vi "User Interface.vi"(10 "Test File Path":path=path "") -> ()   [LabVIEW 2020, in "Execution UI.lvclass"]
uses:
  Execution UI.lvclass
  Execution UI.lvclass/Execution UI.ctl
  Application Framework/Process Classes/Process/Process.lvclass
  <vilib>/Utility/miscctls.llb/LVNodeAndColumnTypeDef.ctl
  Private/TypeDefs/Execution State.ctl
  Framework/Result View/Result View.vi
  Framework/Test Result View/Test Result View.lvclass
  <vilib>/Platform/browser.llb/Open URL in Default Browser (string).vi
  Core/Result/Status.ctl
  Core/Result/Result.lvlib
  Framework/Result Model/Result Model.lvclass
  Core/Result/Type.ctl
  Core/Result/Result.ctl
  109dbbcd-ccfb-4061-a2e5-43f6d68915f9.vi
  C:/Git/astemes-lunit/source/Application Framework/Process Classes/Process/Process.lvclass
  C:/Git/astemes-lunit/source/Execution UI/Execution UI.lvclass
  C:/Git/astemes-lunit/source/Core/Result Observer/Result Observer.lvclass
panel:
  in  "Refresh":bool
  in  "Run Selected Tests":bool
  in  "Stop":bool
  in  "Run All Tests":bool
  in  "Eject":bool
  in  "Save":bool
  in  "Collapse":bool
  in  "Expand":bool
  out "Progress bar":dbl(slide) scale=0.0..100.0
  out "Results":i32(listbox)=-1
  in  "Test Results":string[](tree)
  in  "Filter fails":bool
  out "Description":string
  out "Status":string
  # "1"
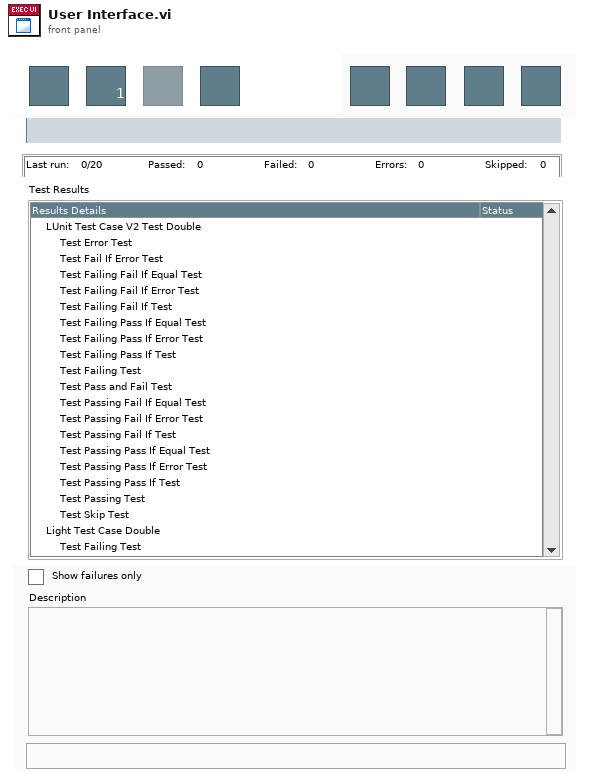
[diagram p1: front panel]
types:
  T1 = typedef "Result Model.lvclass/Statistics.ctl" = cluster{"Method Count":u32, "Executed Methods":u32, "Passed Methods":u32, "Failed Methods":u32, "Method Errors":u32, "Skipped Method":u32, "Progress [%]":dbl}
  T2 = typedef "Execution UI.lvclass/Execution State.ctl" = enum16{"Idle", "Running"}
  T3 = typedef "Result.lvlib/Result.ctl" = cluster{"Name":string, "Message":string, "Description":string, "Status":T4, "Result Type":T5, "Execution Time":dbl}
  T4 = typedef "Result.lvlib/Status.ctl" = enum16{"", "Passed", "Failed", "Error", "Skipped", "Setup Error", "Broken", "Teardown Error"}
  T5 = typedef "Result.lvlib/Type.ctl" = enum16{"Method", "Case", "Suite", "Pass", "Fail", "Skip", "Pass if", "Fail if", "Pass if Error", "Fail if Error", "Pass if Equal", "Fail if Equal"}
  T6 = typedef "LVNodeAndColumnTypeDef.ctl" = cluster{"Node":string, "Column":i32}
  T7 = enum8{"Enabled", "Disabled", "Disabled and Grayed Out"}
  T8 = enum32{"Invalid", "Standard", "Closed", "Hidden", "Minimized", "Maximized"}
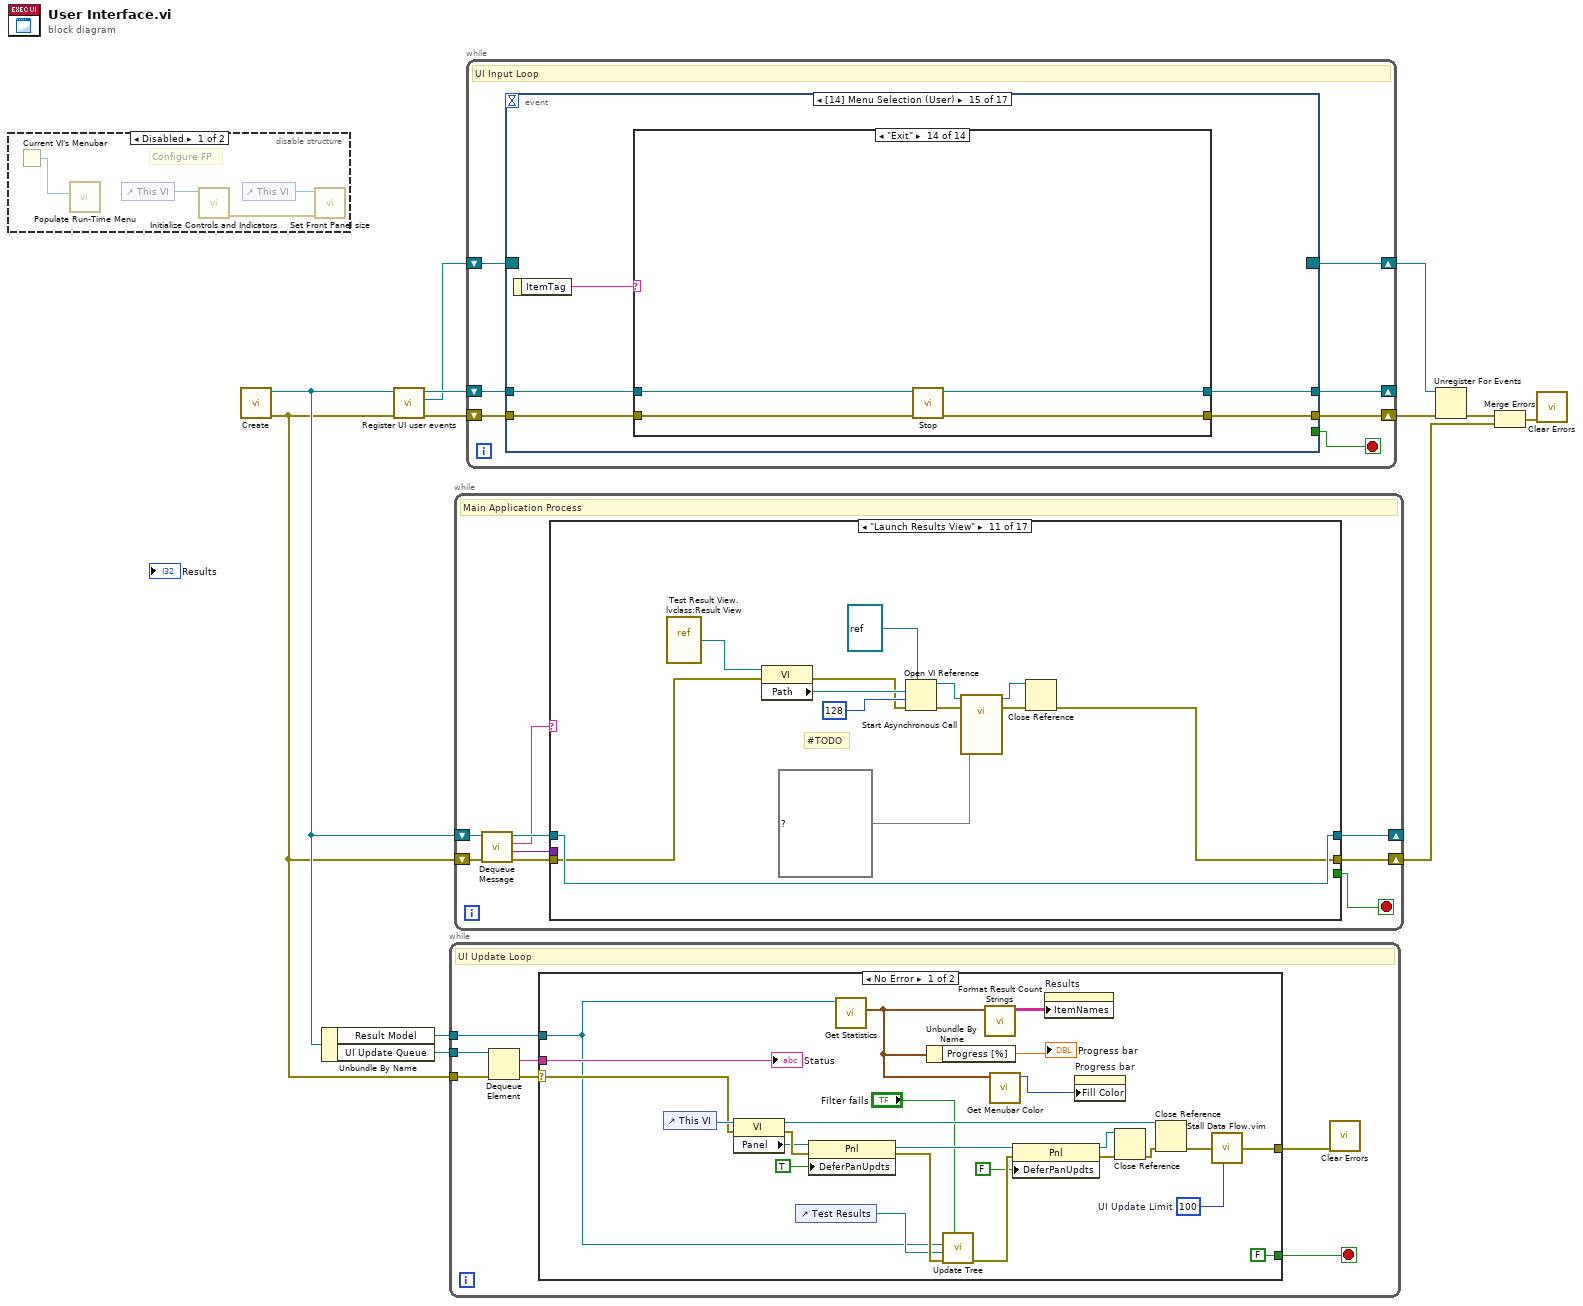
[diagram p0: block diagram]
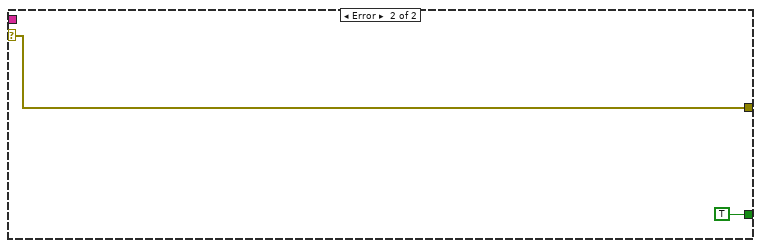
[diagram p2: hidden frame]
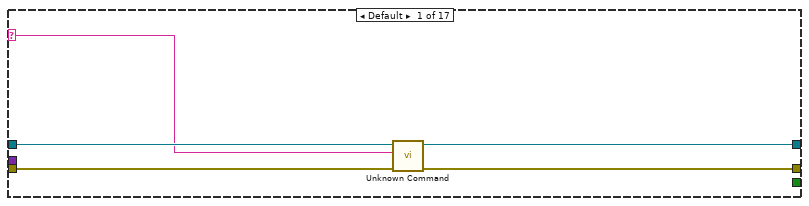
[diagram p3: hidden frame]
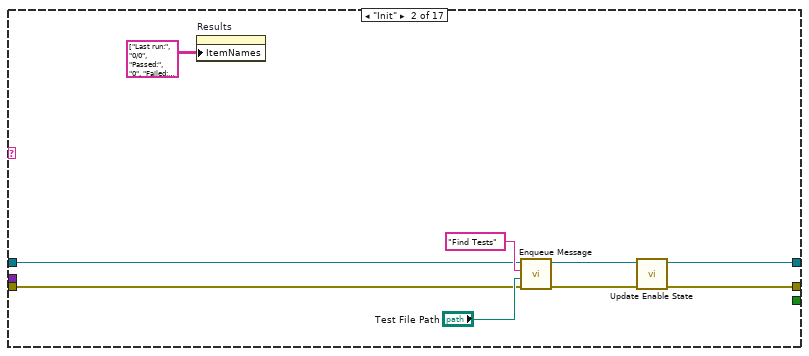
[diagram p4: hidden frame]
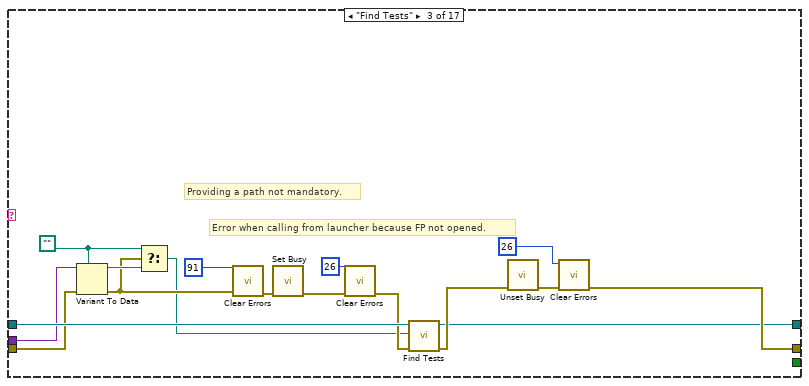
[diagram p5: hidden frame]
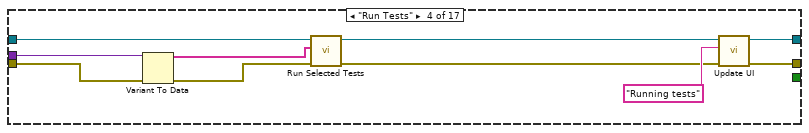
[diagram p6: hidden frame]
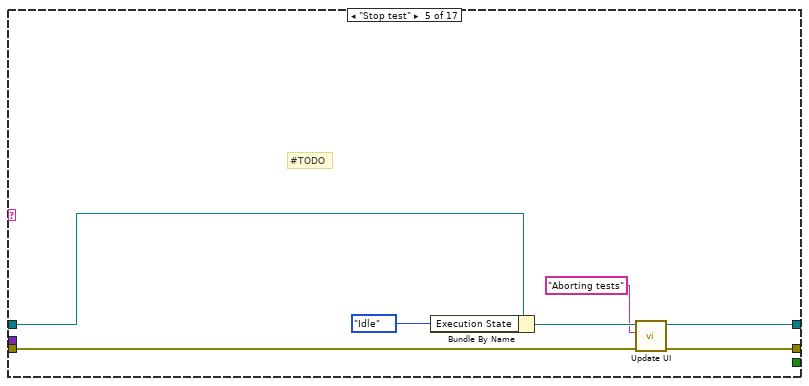
[diagram p7: hidden frame]
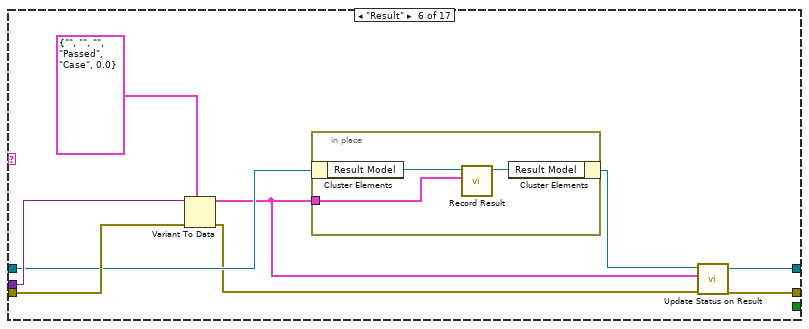
[diagram p8: hidden frame]
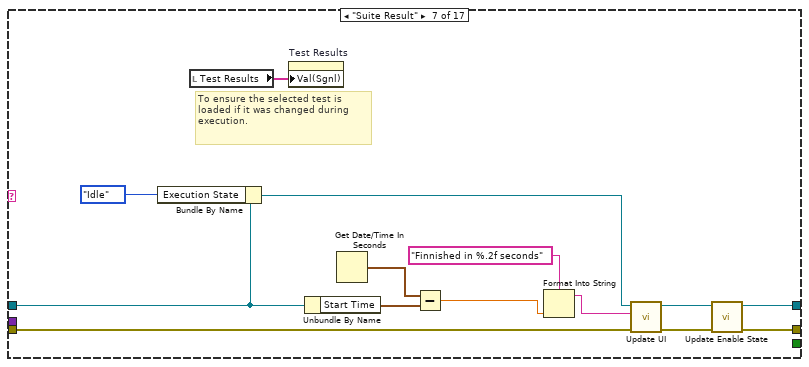
[diagram p9: hidden frame]
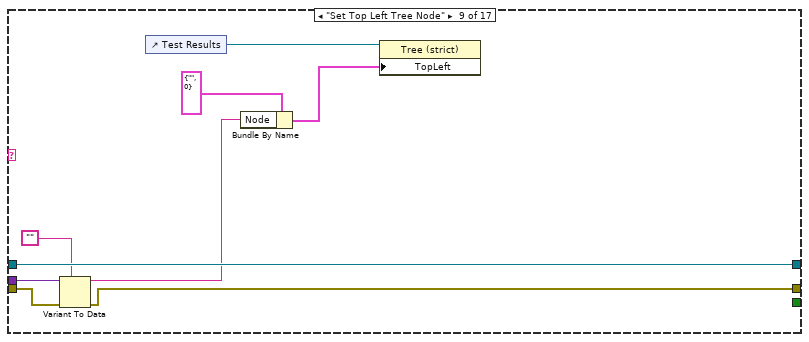
[diagram p11: hidden frame]
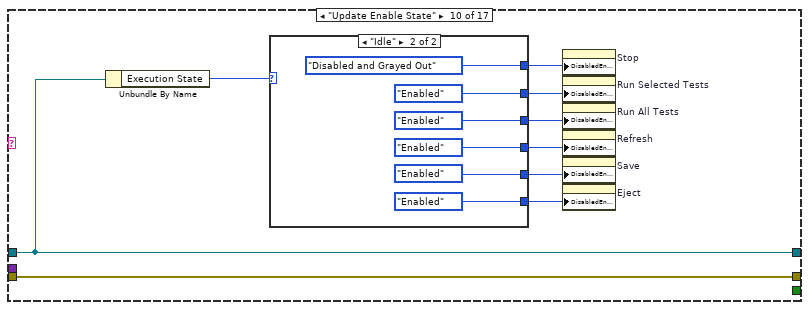
[diagram p12: hidden frame]
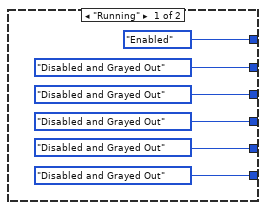
[diagram p13: hidden frame]
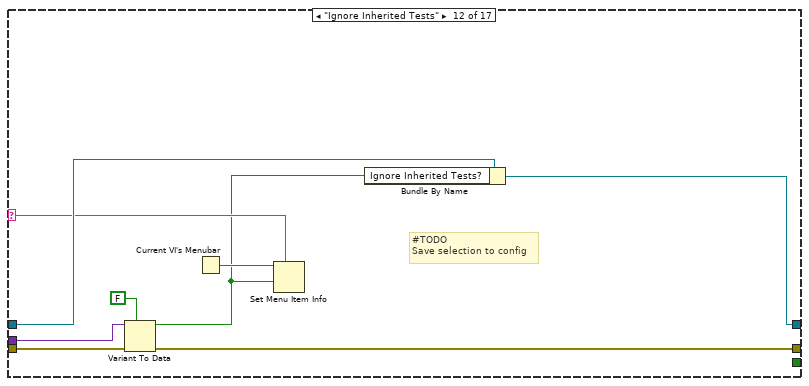
[diagram p14: hidden frame]
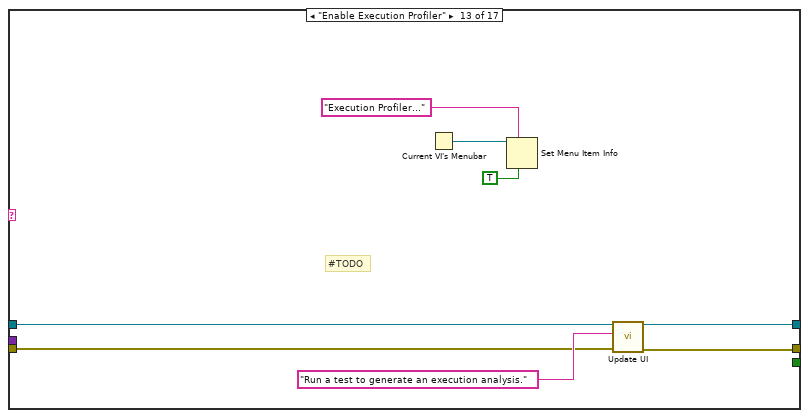
[diagram p15: hidden frame]
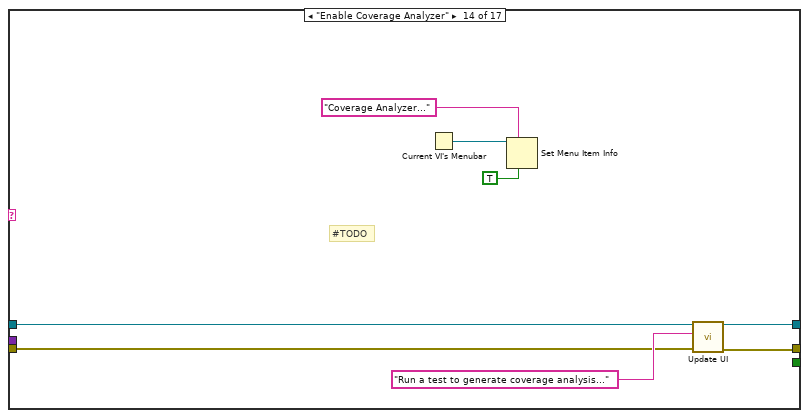
[diagram p16: hidden frame]
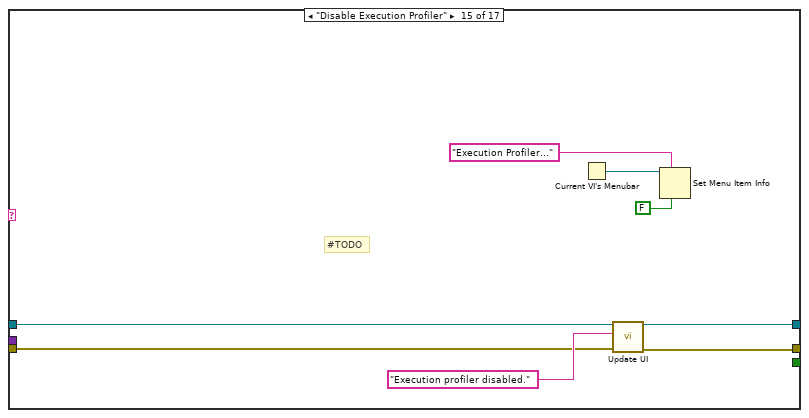
[diagram p17: hidden frame]
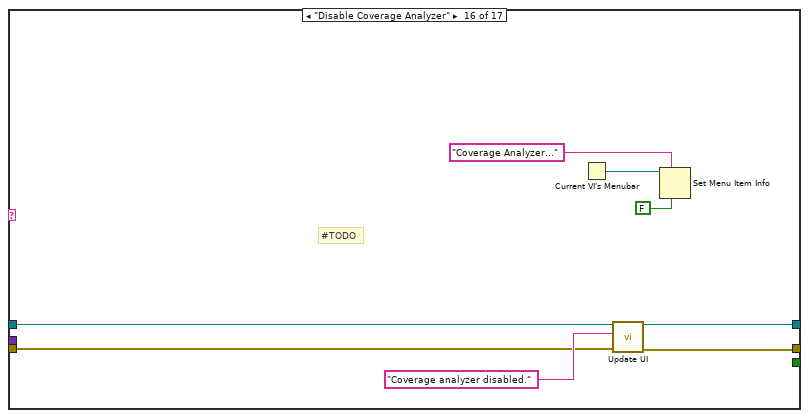
[diagram p18: hidden frame]
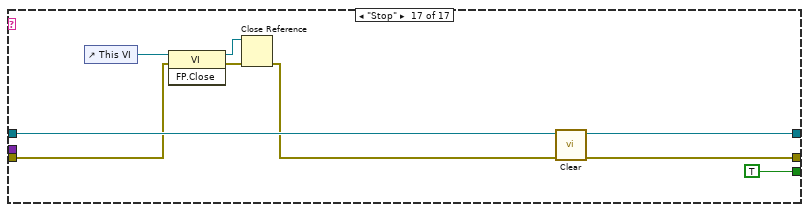
[diagram p19: hidden frame]
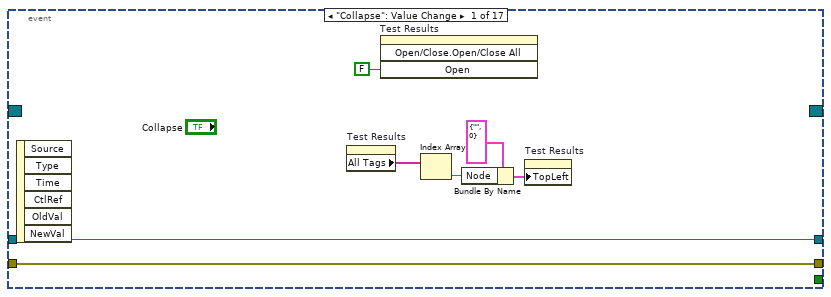
[diagram p20: hidden frame]
diagram:
  n1 = disable-structure shown="Disabled" {
    frame Disabled {
      # "Configure FP"
      n2 = Current VI's Menubar() -> (w13:refnum<k9>)
      n3 = call "Populate Run-Time Menu.vi"("Menu in"=w13) -> ()  [unwired: 9 in, 2 out]
      n4 = control-ref of="This VI"() -> (w15:refnum<vi>)
      n5 = call "Initialize Controls and Indicators.vi"("VI in"=w15) -> ("error out"=w14:errorcluster)  [unwired: 10 in]
      n6 = control-ref of="This VI"() -> (w16:refnum<vi>)
      n7 = call "Set Front Panel size.vi"("error in (no error)"=w14, "VI in"=w16) -> ()  [unwired: 9 in, 1 out]
    }
    frame Enabled {
    }
  }
  n8 = call "Create.vi"() -> ("error out"=w3:errorcluster, "Execution UI Out"=w4:refnum<class "Execution UI.lvclass">)  [unwired: 10 in]
  n9 = Unbundle By Name(w4) -> ("Result Model"=w2:refnum<class "Result Model.lvclass">, "UI Update Queue"=w1:refnum<queue>)
  n10 = call "Register UI user events.vi"("error in (no error)"=w3, "Execution UI In"=w4) -> ("error out"=w11:errorcluster, "Event Registration Refnum"=w9:refnum<event-registration>, "Execution UI Out"=w12:refnum<class "Execution UI.lvclass">)  [unwired: 7 in]
  n11 = while {
    tunnel: w3 -> [w21]
    tunnel: w2 -> [w19]
    tunnel: w1 -> [w18]
    stop <- w17 stop-if-true
    # "UI Update Loop"
    n12 = Dequeue Element(queue=w18, error in (no error)=w21) -> (element=w23:string, error out=w22:errorcluster)  [unwired: 1 in, 2 out]
    n13 = case shown="No Error" w22 {
      selector: w22 -> [w30 w50]
      tunnel: w23 -> [w31 _]
      tunnel: [w28 w50] -> w20
      tunnel: w19 -> [w25 _]
      tunnel: [FALSE TRUE] -> w17
      frame No Error {
        w27 = u32 100  # UI Update Limit
        n14 = control-ref of="This VI"() -> (w37:refnum<vi>)
        n15 = property on="Property Node" class="VI"(reference=w37, error in=w30) -> (reference out=w45:refnum<vi>, error out=w39:errorcluster, "Panel"=w38:refnum<vi>)
        n16 = control-ref of="Test Results"() -> (w32:refnum<vi>)
        n17 = property on="Property Node" class="Pnl"(reference=w38, error in=w39, "DeferPanUpdts"=TRUE ("Defer Panel Updates")) -> (reference out=w44:refnum<vi>, error out=w47:errorcluster)
        n18 = call "Get Statistics.vi"("Result Model in"=w25) -> ("Results"=w36:T1)  [unwired: 10 in]
        n19 = Unbundle By Name(w36) -> ("Progress [%]"=→"Progress bar":dbl)
        n20 = call "Update Tree.vi"("Filter Fails?"="Filter fails", "error in (no error)"=w47, "Test Tree"=w32, "Result Model"=w25) -> ("error out"=w48:errorcluster)  [unwired: 7 in]
        n21 = call "Format Result Count Strings.vi"("Results"=w36) -> ("Array"=w35:string[][])  [unwired: 10 in]
        n22 = call "Get Menubar Color.vi"("Results"=w36) -> ("Fill Color"=w34:u32)  [unwired: 10 in]
        n23 = property on="Property Node" class="Pnl"(reference=w44, error in=w48, "DeferPanUpdts"=FALSE ("Defer Panel Updates")) -> (reference out=w43:refnum<vi>, error out=w41:errorcluster)
        n24 = property on="Results" class="MCListbox (strict)"("ItemNames"=w35) -> ()  [unwired: 2 in, 2 out]
        n25 = property on="Progress bar" class="Slide (strict)"("Fill Color"=w34) -> ()  [unwired: 2 in, 2 out]
        n26 = Close Reference(reference=w43, error in (no error)=w41) -> (error out=w42:errorcluster)
        n27 = Close Reference(reference=w45, error in (no error)=w42) -> (error out=w29:errorcluster)
        n28 = call "Stall Data Flow.vim"("value in"=w29, "milliseconds to wait"=w27) -> ("value out"=w28:errorcluster)  [unwired: 1 out]
        "Status" <- w31
      }
      frame Error {
      }
    }
    n29 = call <vilib>:"Clear Errors.vi"("error in (no error)"=w20) -> ()  [unwired: 5 in, 2 out]
  }
  n30 = while {
    shift-right: [w51] -> w8
    shift-left: w3 -> [w58]
    shift-right: [w52] -> _
    shift-left: w4 -> [w59]
    stop <- w55 stop-if-true
    # "Main Application Process"
    n31 = call "Dequeue Message.vi"("error in (no error)"=w58, "Process In"=w59) -> ("error out"=w56:errorcluster, "Message Data"=w53:variant, "Message"=w54:string, "Process Out"=w57:refnum<class "Execution UI.lvclass">)  [unwired: 6 in]
    n32 = case shown="\"Launch Results View\"" w54 {
      selector: w54 -> [w60 _ _ _ _ _ _ _ _ _ _ w181 _ _ _ _ _]
      tunnel: w57 -> [w61 w66 w90 w94 w106 w113 w123 w135 w143 w152 w178 w187 w194 w202 w210 w218 w225]
      tunnel: [w62 w71 w74 w100 w101 w111 w124 w135 w143 w152 w178 w180 w192 w200 w208 w216 w228] -> w52
      tunnel: w56 -> [w63 w67 w84 w96 w105 w116 w133 w134 w144 w153 w176 w186 w188 w199 w207 w215 w220]
      tunnel: [w64 w70 w77 w99 w104 w109 w126 w134 w140 w153 w177 w185 w193 w201 w209 w217 w227] -> w51
      tunnel: [_ _ _ _ _ _ _ _ _ _ _ _ _ _ _ _ TRUE] -> w55
      tunnel: w53 -> [_ _ w87 w92 _ w114 _ _ w142 _ _ w184 _ _ _ _ _]
      frame Default {
        n33 = call "Unknown Command.vi"("error in (no error)"=w63, "String"=w60, "Process In"=w61) -> ("error out"=w64:errorcluster, "Process Out"=w62:refnum<class "Execution UI.lvclass">)  [unwired: 7 in]
      }
      frame "Init" {
        n34 = property on="Results" class="MCListbox (strict)"("ItemNames"=string[][] [["Last run:", "0/0", "Passed:", "0", "Failed:", "0", "Errors:", "0", "Skipped:", "0"]] ("Result Texts")) -> ()  [unwired: 2 in, 2 out]
        n35 = call "Enqueue Message.vi"("error in (no error)"=w67, "Message Data"="Test File Path", "Message"="Find Tests", "Process In"=w66) -> ("error out"=w72:errorcluster, "Process Out"=w73:refnum<class "Execution UI.lvclass">)  [unwired: 6 in]
        n36 = call "Update Enable State.vi"("error in (no error)"=w72, "Execution UI In"=w73) -> ("error out"=w70:errorcluster, "Execution UI Out"=w71:refnum<class "Execution UI.lvclass">)  [unwired: 8 in]
      }
      frame "Find Tests" {
        w86 = path "" ("Not A Path Constant")
        # "Error when calling from launcher because FP not opened."
        # "Providing a path not mandatory."
        n37 = Variant To Data(error in=w84, type=w86, Variant=w87) -> (data=w85:path, error out=w81:errorcluster)
        n38 = Select(t=w86, s=w81, f=w85) -> (s? t:f=w76:path)
        n39 = call <vilib>:"Clear Errors.vi"("error in (no error)"=w81, "specific error code to clear (0: all)"=91) -> ("error out"=w83:errorcluster)  [unwired: 4 in, 1 out]
        n40 = call <vilib>:"Set Busy.vi"("error in (no error)"=w83) -> ("error out"=w89:errorcluster)  [unwired: 9 in, 1 out]
        n41 = call <vilib>:"Clear Errors.vi"("error in (no error)"=w89, "specific error code to clear (0: all)"=26) -> ("error out"=w80:errorcluster)  [unwired: 4 in, 1 out]
        n42 = call "Find Tests.vi"("error in (no error)"=w80, "Project or Class Path"=w76, "Execution UI In"=w90) -> ("error out"=w75:errorcluster, "Execution UI Out"=w74:refnum<class "Execution UI.lvclass">)  [unwired: 7 in]
        n43 = call <vilib>:"Unset Busy.vi"("error in (no error)"=w75) -> ("error out"=w88:errorcluster)  [unwired: 10 in]
        n44 = call <vilib>:"Clear Errors.vi"("error in (no error)"=w88, "specific error code to clear (0: all)"=26) -> ("error out"=w77:errorcluster)  [unwired: 4 in, 1 out]
      }
      frame "Run Tests" {
        n45 = Variant To Data(error in=w96, Variant=w92) -> (data=w91:string[], error out=w93:errorcluster)  [unwired: 1 in]
        n46 = call "Run Selected Tests.vi"("error in (no error)"=w93, "Tests"=w91, "Execution UI In"=w94) -> ("error out"=w97:errorcluster, "Execution UI Out"=w95:refnum<class "Execution UI.lvclass">)  [unwired: 7 in]
        n47 = call "Update UI.vi"("error in (no error)"=w97, "Status"="Running tests", "Execution UI In"=w95) -> ("error out"=w99:errorcluster, "Execution UI Out"=w100:refnum<class "Execution UI.lvclass">)  [unwired: 7 in]
      }
      frame "Stop test" {
        # "#TODO"
        n48 = Bundle By Name(cluster=w106, "Execution State"=Execution_State."Idle") -> (w107:refnum<class "Execution UI.lvclass">)
        n49 = call "Update UI.vi"("error in (no error)"=w105, "Status"="Aborting tests", "Execution UI In"=w107) -> ("error out"=w104:errorcluster, "Execution UI Out"=w101:refnum<class "Execution UI.lvclass">)  [unwired: 7 in]
      }
      frame "Result" {
        n50 = Variant To Data(error in=w116, type=T3 {"Name"="", "Message"="", "Description"="", "Status"=enum."Passed", "Result Type"=enum."Case", "Execution Time"=0.0} ("Result"), Variant=w114) -> (data=w108:T3, error out=w110:errorcluster)
        n51 = in-place {
          in-place-border: w108 -> [w119]
          n52 = in-place-cluster #1(w113) -> ("Result Model"=w118:refnum<class "Result Model.lvclass">)
          n53 = call "Record Result.vi"("Results"=w119, "Result Model in"=w118) -> ("Result Model out"=w117:refnum<class "Result Model.lvclass">)  [unwired: 9 in]
          n54 = in-place-cluster #1("Result Model"=w117) -> (w112:refnum<class "Execution UI.lvclass">)
        }
        n55 = call "Update Status on Result.vi"("error in (no error)"=w110, "Result"=w108, "Execution UI V2 in"=w112) -> ("error out"=w109:errorcluster, "Execution UI V2 out"=w111:refnum<class "Execution UI.lvclass">)  [unwired: 7 in]
      }
      frame "Suite Result" {
        # "To ensure the selected test is loaded if it was changed during execution."
        n56 = Bundle By Name(cluster=w123, "Execution State"=Execution_State."Idle") -> (w129:refnum<class "Execution UI.lvclass">)
        n57 = local read "Test Results"() -> (w127:string[])
        n58 = property on="Test Results" class="Tree (strict)"("Val(Sgnl)"=w127) -> ()  [unwired: 2 in, 2 out]
        n59 = Unbundle By Name(w123) -> ("Start Time"=w121:timestamp)
        n60 = Get Date/Time In Seconds() -> (seconds since 1Jan1904=w122:timestamp)
        n61 = Subtract(x=w122, y=w121) -> (x-y=w120:dbl)
        n62 = Format Into String(format string="Finnished in %.2f seconds", w120) -> (resulting string=w130:string)  [unwired: 2 in, 1 out]
        n63 = call "Update UI.vi"("error in (no error)"=w133, "Status"=w130, "Execution UI In"=w129) -> ("error out"=w132:errorcluster, "Execution UI Out"=w125:refnum<class "Execution UI.lvclass">)  [unwired: 7 in]
        n64 = call "Update Enable State.vi"("error in (no error)"=w132, "Execution UI In"=w125) -> ("error out"=w126:errorcluster, "Execution UI Out"=w124:refnum<class "Execution UI.lvclass">)  [unwired: 8 in]
      }
      frame "Save results" {
        # "#TODO"
      }
      frame "Set Top Left Tree Node" {
        n65 = Variant To Data(error in=w144, type="", Variant=w142) -> (data=w136:string, error out=w140:errorcluster)
        n66 = control-ref of="Test Results"() -> (w139:refnum<vi>)
        n67 = Bundle By Name(cluster=T6 {"Node"="", "Column"=0} ("Top Left Visible Cell"), "Node"=w136) -> (w137:T6)
        n68 = property on="Property Node" class="Tree (strict)"(reference=w139, "TopLeft"=w137) -> ()  [unwired: 1 in, 2 out]
      }
      frame "Update Enable State" {
        n69 = Unbundle By Name(w152) -> ("Execution State"=w151:T2)
        n70 = case shown="\"Idle\"" w151 {
          tunnel: [T7."Enabled" ("Disabled") T7."Disabled and Grayed Out" ("Disabled")] -> w150
          tunnel: [T7."Disabled and Grayed Out" ("Disabled") T7."Enabled" ("Disabled")] -> w149
          tunnel: [T7."Disabled and Grayed Out" ("Disabled") T7."Enabled" ("Disabled")] -> w148
          tunnel: [T7."Disabled and Grayed Out" ("Disabled") T7."Enabled" ("Disabled")] -> w147
          tunnel: [T7."Disabled and Grayed Out" ("Disabled") T7."Enabled" ("Disabled")] -> w146
          tunnel: [T7."Disabled and Grayed Out" ("Disabled") T7."Enabled" ("Disabled")] -> w145
          frame "Running" {
          }
          frame "Idle" {
          }
        }
        n71 = property on="Stop" class="Bool"("DisabledEnum"=w150) -> ()  [unwired: 2 in, 2 out]
        n72 = property on="Run Selected Tests" class="Bool"("DisabledEnum"=w149) -> ()  [unwired: 2 in, 2 out]
        n73 = property on="Run All Tests" class="Bool"("DisabledEnum"=w148) -> ()  [unwired: 2 in, 2 out]
        n74 = property on="Refresh" class="Bool"("DisabledEnum"=w147) -> ()  [unwired: 2 in, 2 out]
        n75 = property on="Save" class="Bool"("DisabledEnum"=w146) -> ()  [unwired: 2 in, 2 out]
        n76 = property on="Eject" class="Bool"("DisabledEnum"=w145) -> ()  [unwired: 2 in, 2 out]
      }
      frame "Launch Results View" {
        # "#TODO"
        n77 = vi-ref "Test Result View.lvclass:Result View.vi"() -> (w173:refnum<vi>)
        n78 = property class="VI"(reference=w173, error in=w176) -> (error out=w168:errorcluster, "Path"=w172:path)  [unwired: 1 out]
        n79 = Open VI Reference(type specifier VI Refnum (for type only)=refnum<vi> refnum, vi path=w172, options=128, error in (no error)=w168) -> (vi reference=w169:refnum<vi>, error out=w171:errorcluster)  [unwired: 2 in]
        n80 = call-by-ref "Start Asynchronous Call"(reference=w169, error in=w171, "TestCase map"=map{string, map{string, path}} {}) -> (reference out=w174:refnum<vi>, error out=w175:errorcluster)  [unwired: 11 in]
        n81 = Close Reference(reference=w174, error in (no error)=w175) -> (error out=w177:errorcluster)
      }
      frame "Ignore Inherited Tests" {
        # "#TODO \nSave selection to config"
        n82 = Variant To Data(error in=w186, type=FALSE, Variant=w184) -> (data=w179:bool, error out=w185:errorcluster)
        n83 = Current VI's Menubar() -> (w182:refnum<k9>)
        n84 = Set Menu Item Info(7:w181, 9:w179, 11:w182) -> ()  [unwired: 4 in, 2 out]
        n85 = Bundle By Name(cluster=w187, "Ignore Inherited Tests?"=w179) -> (w180:refnum<class "Execution UI.lvclass">)
      }
      frame "Enable Execution Profiler" {
        # "#TODO"
        n86 = Current VI's Menubar() -> (w191:refnum<k9>)
        n87 = Set Menu Item Info(6:TRUE ("checked"), 7:"Execution Profiler...", 11:w191) -> ()  [unwired: 4 in, 2 out]
        n88 = call "Update UI.vi"("error in (no error)"=w188, "Status"="Run a test to generate an execution analysis.", "Execution UI In"=w194) -> ("error out"=w193:errorcluster, "Execution UI Out"=w192:refnum<class "Execution UI.lvclass">)  [unwired: 7 in]
      }
      frame "Enable Coverage Analyzer" {
        # "#TODO"
        n89 = Current VI's Menubar() -> (w198:refnum<k9>)
        n90 = Set Menu Item Info(6:TRUE ("checked"), 7:"Coverage Analyzer...", 11:w198) -> ()  [unwired: 4 in, 2 out]
        n91 = call "Update UI.vi"("error in (no error)"=w199, "Status"="Run a test to generate coverage analysis...", "Execution UI In"=w202) -> ("error out"=w201:errorcluster, "Execution UI Out"=w200:refnum<class "Execution UI.lvclass">)  [unwired: 7 in]
      }
      frame "Disable Execution Profiler" {
        # "#TODO"
        n92 = Current VI's Menubar() -> (w206:refnum<k9>)
        n93 = call "Update UI.vi"("error in (no error)"=w207, "Status"="Execution profiler disabled.", "Execution UI In"=w210) -> ("error out"=w209:errorcluster, "Execution UI Out"=w208:refnum<class "Execution UI.lvclass">)  [unwired: 7 in]
        n94 = Set Menu Item Info(6:FALSE ("checked"), 7:"Execution Profiler...", 11:w206) -> ()  [unwired: 4 in, 2 out]
      }
      frame "Disable Coverage Analyzer" {
        # "#TODO"
        n95 = Current VI's Menubar() -> (w214:refnum<k9>)
        n96 = call "Update UI.vi"("error in (no error)"=w215, "Status"="Coverage analyzer disabled.", "Execution UI In"=w218) -> ("error out"=w217:errorcluster, "Execution UI Out"=w216:refnum<class "Execution UI.lvclass">)  [unwired: 7 in]
        n97 = Set Menu Item Info(6:FALSE ("checked"), 7:"Coverage Analyzer...", 11:w214) -> ()  [unwired: 4 in, 2 out]
      }
      frame "Stop" {
        n98 = control-ref of="This VI"() -> (w224:refnum<vi>)
        n99 = invoke on="Invoke Node" class="VI" method="FP.Close"(reference=w224, error in=w220) -> (reference out=w222:refnum<vi>, error out=w223:errorcluster)  [unwired: 1 in, 1 out]
        n100 = Close Reference(reference=w222, error in (no error)=w223) -> (error out=w221:errorcluster)
        n101 = call-dynamic "Clear.vi"("error in (no error)"=w221, "Execution UI In"=w225) -> ("error out"=w227:errorcluster, "Execution UI Out"=w228:refnum<class "Execution UI.lvclass">)  [unwired: 8 in]
      }
    }
  }
  n102 = while {
    shift-right: [w229] -> w7
    shift-left: w11 -> [w234]
    shift-right: [w230] -> _
    shift-left: w12 -> [w235]
    shift-right: [w232] -> w10
    shift-left: w9 -> [w231]
    stop <- w233 stop-if-true
    # "UI Input Loop"
    n103 = event shown="[14] Menu Selection (User)" {
      selector: w231 -> [_ _ _ _ _ _ _ _ _ _ _ _ _ _ _ _ _]
      dyn-events: [_ _ _ _ _ _ _ _ _ _ _ _ _ _ _ _ _] -> w232
      timeout: _ -> [_ _ _ _ _ _ _ _ _ _ _ _ _ _ _ _ _]
      tunnel: w235 -> [w241 w244 w249 w257 w261 w274 w300 w307 w318 w323 w327 w329 w349 w357 w392 w500 w506]
      tunnel: w234 -> [w242 w245 w247 w258 w263 w275 w302 w310 w317 w321 w325 w334 w339 w350 w391 w501 w503]
      tunnel: [w242 w245 w248 w256 w264 w273 w299 w306 w317 w320 w326 w334 w340 w355 w390 w501 w504] -> w229
      tunnel: [w241 w244 w250 w254 w262 w272 w297 w304 w318 w322 w328 w329 w349 w354 w389 w500 w505] -> w230
      tunnel: [_ _ _ _ _ _ _ _ _ _ _ _ _ _ _ TRUE _] -> w233
      event "Collapse": Value Change {
        n104 = event-data() -> ()  [unwired: 1 in, 6 out]
        n105 = property on="Test Results" class="Tree (strict)"() -> ("All Tags"=w239:string[])  [unwired: 2 in, 2 out]
        n106 = invoke on="Test Results" class="Tree (strict)" method="Open/Close.Open/Close All"("Open"=FALSE ("Open?")) -> ()  [unwired: 3 in, 4 out]
        n107 = Index Array(array=w239) -> (element=w236:string)  [unwired: 1 in]
        n108 = Bundle By Name(cluster=T6 {"Node"="", "Column"=0} ("Top Left Visible Cell"), "Node"=w236) -> (w237:T6)
        n109 = property on="Test Results" class="Tree (strict)"("TopLeft"=w237) -> ()  [unwired: 2 in, 2 out]
      }
      event "Expand": Value Change {
        n110 = event-data() -> ()  [unwired: 1 in, 6 out]
        n111 = invoke on="Test Results" class="Tree (strict)" method="Open/Close.Open/Close All"("Open"=TRUE ("Open?")) -> ()  [unwired: 3 in, 4 out]
      }
      event "Refresh": Value Change {
        # "#TODO"
        n112 = event-data() -> ()  [unwired: 1 in, 1 out]
        n113 = call "Update UI.vi"("error in (no error)"=w247, "Status"="Recreating test case index.. ", "Execution UI In"=w249) -> ("error out"=w248:errorcluster, "Execution UI Out"=w250:refnum<class "Execution UI.lvclass">)  [unwired: 7 in]
        n114 = One Button Dialog(message="To do") -> ()  [unwired: 1 in, 1 out]
      }
      event "Run All Tests": Value Change {
        n115 = event-data() -> ()  [unwired: 1 in, 1 out]
        n116 = call "Enqueue Message.vi"("error in (no error)"=w258, "Message Data"=string[] [] ("data"), "Message"="Run Tests", "Process In"=w257) -> ("error out"=w259:errorcluster, "Process Out"=w255:refnum<class "Execution UI.lvclass">)  [unwired: 6 in]
        n117 = call "Update Enable State.vi"("error in (no error)"=w259, "Execution UI In"=w255) -> ("error out"=w256:errorcluster, "Execution UI Out"=w254:refnum<class "Execution UI.lvclass">)  [unwired: 8 in]
      }
      event "Filter fails": Value Change {
        n118 = event-data() -> ("NewVal"=w260:bool)  [unwired: 1 in]
        n119 = Select(t="Showing only failed tests", s=w260, f="Showing all tests") -> (s? t:f=w267:string)
        n120 = call "Update UI.vi"("error in (no error)"=w263, "Status"=w267, "Execution UI In"=w261) -> ("error out"=w264:errorcluster, "Execution UI Out"=w262:refnum<class "Execution UI.lvclass">)  [unwired: 7 in]
      }
      event Key Down {
        # "Run all tests on ctrl+r"
        n121 = event-data() -> ("Char"=w268:i16, "PlatMods.Ctrl"=w271:bool, "PlatMods.Opt"=w270:bool)  [unwired: 1 in]
        n122 = Or(x=w271, y=w270) -> (x .or. y?=w269:bool)
        n123 = case "CTRL" shown="True" w269 {
          tunnel: w275 -> [w276 w282]
          tunnel: w274 -> [w277 w281]
          tunnel: [w276 w280] -> w273
          tunnel: [w277 w279] -> w272
          tunnel: w268 -> [_ w278]
          frame False {
          }
          frame True {
            n124 = case "Key" shown="119" w278 {
              tunnel: w282 -> [w283 w290 w294]
              tunnel: w281 -> [w284 w288 w295]
              tunnel: [w283 w287 w292] -> w280
              tunnel: [w284 w285 w293] -> w279
              frame Default {
              }
              frame 114 {
                w289 = "Run all tests"  # Message
                # "R"
                n125 = call "Enqueue Message.vi"("error in (no error)"=w290, "Message"=w289, "Process In"=w288) -> ("error out"=w291:errorcluster, "Process Out"=w286:refnum<class "Execution UI.lvclass">)  [unwired: 7 in]
                n126 = call "Update Enable State.vi"("error in (no error)"=w291, "Execution UI In"=w286) -> ("error out"=w287:errorcluster, "Execution UI Out"=w285:refnum<class "Execution UI.lvclass">)  [unwired: 8 in]
              }
              frame 119 {
                # "W"
                n127 = call-dynamic "Stop.vi"("error in (no error)"=w294, "Execution UI In"=w295) -> ("error out"=w292:errorcluster, "Execution UI Out"=w293:refnum<class "Execution UI.lvclass">)  [unwired: 8 in]
              }
            }
          }
        }
      }
      event "Run Selected Tests": Value Change {
        # "#TODO"
        n128 = event-data() -> ()  [unwired: 1 in, 1 out]
        n129 = call "Enqueue Message.vi"("error in (no error)"=w302, "Message Data"="Test Results", "Message"="Run Tests", "Process In"=w300) -> ("error out"=w303:errorcluster, "Process Out"=w298:refnum<class "Execution UI.lvclass">)  [unwired: 6 in]
        n130 = call "Update Enable State.vi"("error in (no error)"=w303, "Execution UI In"=w298) -> ("error out"=w299:errorcluster, "Execution UI Out"=w297:refnum<class "Execution UI.lvclass">)  [unwired: 8 in]
      }
      event "Stop": Value Change {
        n131 = event-data() -> ()  [unwired: 1 in, 2 out]
        n132 = call "Enqueue Message.vi"("error in (no error)"=w310, "Message"="Stop test", "Process In"=w307) -> ("error out"=w309:errorcluster, "Process Out"=w305:refnum<class "Execution UI.lvclass">)  [unwired: 7 in]
        n133 = call "Update Enable State.vi"("error in (no error)"=w309, "Execution UI In"=w305) -> ("error out"=w306:errorcluster, "Execution UI Out"=w304:refnum<class "Execution UI.lvclass">)  [unwired: 8 in]
      }
      event "Test Results": Double Click {
        n134 = event-data() -> ("Tag"=w311:string)  [unwired: 1 in]
        n135 = Open VI Reference(vi path=w311) -> (vi reference=w312:refnum<vi>, error out=w313:errorcluster)  [unwired: 5 in]
        n136 = invoke class="VI" method="FP.Open"(reference=w312, error in=w313) -> (reference out=w315:refnum<vi>, error out=w314:errorcluster)  [unwired: 3 in, 3 out]
        n137 = Close Reference(reference=w315, error in (no error)=w314) -> (error out=w316:errorcluster)
        n138 = call <vilib>:"Clear Errors.vi"("error in (no error)"=w316) -> ()  [unwired: 5 in, 2 out]
      }
      event "Save": Value Change {
        n139 = event-data() -> ()  [unwired: 1 in, 1 out]
        n140 = call "Enqueue Message.vi"("error in (no error)"=w321, "Message"="Save results", "Process In"=w323) -> ("error out"=w320:errorcluster, "Process Out"=w322:refnum<class "Execution UI.lvclass">)  [unwired: 7 in]
      }
      event "Eject": Value Change {
        n141 = event-data() -> ()  [unwired: 1 in, 4 out]
        n142 = call "Enqueue Message.vi"("error in (no error)"=w325, "Message"="Launch Results View", "Process In"=w327) -> ("error out"=w326:errorcluster, "Process Out"=w328:refnum<class "Execution UI.lvclass">)  [unwired: 7 in]
      }
      event "Test Results": Value Change {
        n143 = event-data() -> ("NewVal"=w330:string[])  [unwired: 1 in]
        n144 = for {
          tunnel: w329 -> [w338]
          tunnel: w330 -> [w336] mode=indexing
          tunnel: [w335] -> w332 mode=indexing
          n145 = Unbundle By Name(w338) -> ("Result Model"=w337:refnum<class "Result Model.lvclass">)
          n146 = call "Get Summary.vi"("Item"=w336, "Result Model In"=w337) -> ("Summary"=w335:string)  [unwired: 9 in]
        }
        n147 = call <vilib>:"1D String Array to Delimited String.vi"("delimiter"="\n", "string array"=w332) -> ("delimited string"=→"Description":string)  [unwired: 9 in]
      }
      event Pane Size {
        # "Set column sizes on pane resize."
        n148 = event-data() -> ()  [unwired: 1 in, 1 out]
        n149 = property on="Test Results" class="Tree (strict)"(error in=w339) -> (error out=w341:errorcluster, "Width"=w342:u32)  [unwired: 1 in, 1 out]
        n150 = Quotient & Remainder(x=w342, y=u32 10) -> (floor(x/y)=w346:u32)  [unwired: 1 out]
        n151 = Multiply(x=w346, y=u32 8) -> (x*y=w343:u32)
        n152 = property on="Test Results" class="Tree (strict)"(error in=w341, "ActiveColNum"=0 ("Active Cell:Active Column Number"), "Width"=w343, "ActiveColNum"=1 ("Active Cell:Active Column Number"), "Width"=w343) -> (error out=w340:errorcluster)  [unwired: 1 in, 1 out]
      }
      event "Test File Path": Value Change {
        # "#TODO"
        # "This case is triggered when running test cases through VI Server.\nTo control test execution from an external VI - get a reference to the \"Test File Path\" control on the User Interface.vi and update the value with the path to test case using a property node."
        n153 = event-data() -> ("NewVal"=w356:path)  [unwired: 1 in]
        n154 = call <vilib>:"Get File Extension.vi"("error in (no error)"=w350, "file"=w356) -> ("error out"=w351:errorcluster, "lowercase file extension"=w352:string, "dup file"=w353:path)  [unwired: 5 in, 2 out]
        n155 = case shown="\"lvclass\"" w352 {
          tunnel: w357 -> [w359 w378 w387]
          tunnel: w351 -> [w358 w377 w386]
          tunnel: w353 -> [_ w372 w384]
          tunnel: [w358 w364 w381] -> w355
          tunnel: [w359 w362 w380] -> w354
          frame Default {
          }
          frame "lvclass" {
            n156 = call "Enqueue Message.vi"("error in (no error)"=w377, "Message Data"=w372, "Message"="Find Tests", "Process In"=w378) -> ("error out"=w368:errorcluster, "Process Out"=w370:refnum<class "Execution UI.lvclass">)  [unwired: 6 in]
            n157 = call <vilib>:"Get LV Class Default Value.vi"("error in (no error)"=w368, "class path"=w372) -> ("error out"=w374:errorcluster, "object"=w373:refnum<class>)  [unwired: 8 in]
            n158 = call <vilib>:"Get LV Class Name.vi"("error in (no error)"=w374, "object"=w373) -> ("error out"=w367:errorcluster, "class name"=w361:string)  [unwired: 8 in]
            n159 = Build Array(w361) -> (w366:string[])
            n160 = call "Enqueue Message.vi"("error in (no error)"=w367, "Message Data"=w366, "Message"="Select Tests", "Process In"=w370) -> ("error out"=w371:errorcluster, "Process Out"=w369:refnum<class "Execution UI.lvclass">)  [unwired: 6 in]
            n161 = call "Enqueue Message.vi"("error in (no error)"=w371, "Message"="Run Selected Tests", "Process In"=w369) -> ("error out"=w365:errorcluster, "Process Out"=w363:refnum<class "Execution UI.lvclass">)  [unwired: 7 in]
            n162 = call "Enqueue Message.vi"("error in (no error)"=w365, "Message Data"=w361, "Message"="Set Top Left Tree Node", "Process In"=w363) -> ("error out"=w364:errorcluster, "Process Out"=w362:refnum<class "Execution UI.lvclass">)  [unwired: 6 in]
          }
          frame "lvproj" {
            n163 = call "Enqueue Message.vi"("error in (no error)"=w386, "Message Data"=w384, "Message"="Find Tests", "Process In"=w387) -> ("error out"=w382:errorcluster, "Process Out"=w383:refnum<class "Execution UI.lvclass">)  [unwired: 6 in]
            n164 = call "Enqueue Message.vi"("error in (no error)"=w382, "Message"="Run all tests", "Process In"=w383) -> ("error out"=w381:errorcluster, "Process Out"=w380:refnum<class "Execution UI.lvclass">)  [unwired: 7 in]
          }
        }
      }
      event Menu Selection (User) {
        n165 = event-data() -> ("ItemTag"=w393:string)  [unwired: 1 in]
        n166 = case shown="\"Exit\"" w393 {
          tunnel: w392 -> [w407 w409 w416 w424 w437 w440 w448 w465 w478 w485 w489 w493 w494 w499]
          tunnel: w391 -> [w394 w408 w413 w425 w438 w441 w445 w462 w480 w482 w486 w490 w495 w498]
          tunnel: [w395 w408 w411 w426 w438 w441 w446 w463 w479 w483 w487 w491 w495 w497] -> w390
          tunnel: [w407 w409 w412 w427 w437 w440 w447 w464 w478 w485 w489 w493 w494 w496] -> w389
          frame "Full size" {
            # "This is the same as done in event case for Result Pane: Pane Size, but that case is not trigerd on maximizing window."
            n167 = control-ref of="This VI"() -> (w406:refnum<vi>)
            n168 = property on="Property Node" class="VI"(reference=w406, error in=w394, "FP.State"=T8."Maximized" ("Front Panel Window:State")) -> (error out=w397:errorcluster)  [unwired: 1 out]
            n169 = property on="Test Results" class="Tree (strict)"(error in=w397) -> (error out=w396:errorcluster, "Width"=w404:u32)  [unwired: 1 in, 1 out]
            n170 = Quotient & Remainder(x=w404, y=u32 10) -> (floor(x/y)=w403:u32)  [unwired: 1 out]
            n171 = Multiply(x=w403, y=u32 7) -> (x*y=w402:u32)
            n172 = property on="Test Results" class="Tree (strict)"(error in=w396, "ActiveColNum"=0 ("Active Cell:Active Column Number"), "Width"=w402, "ActiveColNum"=1 ("Active Cell:Active Column Number"), "Width"=w402) -> (error out=w395:errorcluster)  [unwired: 1 in, 1 out]
          }
          frame Default {
          }
          frame "Ignore Inherited Tests" {
            w415 = "Ignore Inherited Tests"
            n173 = Current VI's Menubar() -> (w417:refnum<k9>)
            n174 = Get Menu Item Info(7:w415, 11:w417) -> (4:w414:bool)  [unwired: 1 in, 6 out]
            n175 = Not(x=w414) -> (.not. x?=w410:bool)
            n176 = call "Enqueue Message.vi"("error in (no error)"=w413, "Message Data"=w410, "Message"=w415, "Process In"=w416) -> ("error out"=w411:errorcluster, "Process Out"=w412:refnum<class "Execution UI.lvclass">)  [unwired: 6 in]
          }
          frame "Open Project or Test class" {
            n177 = call "File Dialog"("prompt"="Please select a test class or project file to load.", "pattern (all files)"="*.lvclass;*.lvproj;*.lvlib", "pattern label"="Project or class") -> ("selected path"=w423:path, "cancelled"=w419:bool, "error out"=w418:errorcluster)  [unwired: 9 in, 1 out]
            n178 = call <vilib>:"Clear Errors.vi"("error in (no error)"=w418) -> ()  [unwired: 5 in, 2 out]
            n179 = case shown="False" w419 {
              tunnel: [w429 w435] -> w427
              tunnel: [w428 w434] -> w426
              tunnel: w425 -> [w428 w433]
              tunnel: w424 -> [w429 w432]
              tunnel: w423 -> [_ w431]
              frame True {
              }
              frame False {
                n180 = call "Enqueue Message.vi"("error in (no error)"=w433, "Message Data"=w431, "Message"="Find Tests", "Process In"=w432) -> ("error out"=w434:errorcluster, "Process Out"=w435:refnum<class "Execution UI.lvclass">)  [unwired: 6 in]
              }
            }
          }
          frame "Configure Test Runner" {
            # "#TODO"
            n181 = One Button Dialog(message="TODO") -> ()  [unwired: 1 in, 1 out]
          }
          frame "Configure Reporting" {
            # "#TODO"
            n182 = One Button Dialog(message="TODO") -> ()  [unwired: 1 in, 1 out]
          }
          frame "Execution Profiler..." {
            n183 = Current VI's Menubar() -> (w443:refnum<k9>)
            n184 = Get Menu Item Info(7:"Execution Profiler...", 11:w443) -> (4:w444:bool)  [unwired: 1 in, 6 out]
            n185 = case shown="False" w444 {
              tunnel: w448 -> [w453 w458]
              tunnel: [w452 w457] -> w447
              tunnel: [w451 w456] -> w446
              tunnel: w445 -> [w450 w455]
              frame False {
                n186 = call "Enqueue Message.vi"("error in (no error)"=w450, "Message"="Enable Execution Profiler", "Process In"=w453) -> ("error out"=w451:errorcluster, "Process Out"=w452:refnum<class "Execution UI.lvclass">)  [unwired: 7 in]
              }
              frame True {
                n187 = call "Enqueue Message.vi"("error in (no error)"=w455, "Message"="Disable Execution Profiler", "Process In"=w458) -> ("error out"=w456:errorcluster, "Process Out"=w457:refnum<class "Execution UI.lvclass">)  [unwired: 7 in]
              }
            }
          }
          frame "Coverage Analyzer..." {
            n188 = Current VI's Menubar() -> (w460:refnum<k9>)
            n189 = Get Menu Item Info(7:"Coverage Analyzer...", 11:w460) -> (4:w461:bool)  [unwired: 1 in, 6 out]
            n190 = case shown="True" w461 {
              tunnel: w465 -> [w470 w475]
              tunnel: [w469 w474] -> w464
              tunnel: [w468 w473] -> w463
              tunnel: w462 -> [w467 w472]
              frame False {
                n191 = call "Enqueue Message.vi"("error in (no error)"=w467, "Message"="Enable Coverage Analyzer", "Process In"=w470) -> ("error out"=w468:errorcluster, "Process Out"=w469:refnum<class "Execution UI.lvclass">)  [unwired: 7 in]
              }
              frame True {
                n192 = call "Enqueue Message.vi"("error in (no error)"=w472, "Message"="Disable Coverage Analyzer", "Process In"=w475) -> ("error out"=w473:errorcluster, "Process Out"=w474:refnum<class "Execution UI.lvclass">)  [unwired: 7 in]
              }
            }
          }
          frame "Reset..." {
            n193 = control-ref of="This VI"() -> (w476:refnum<vi>)
            n194 = call "Initialize Controls and Indicators.vi"("error in (no error)"=w480, "VI in"=w476) -> ("error out"=w481:errorcluster)  [unwired: 9 in]
            n195 = control-ref of="This VI"() -> (w477:refnum<vi>)
            n196 = call "Set Front Panel size.vi"("error in (no error)"=w481, "VI in"=w477) -> ("error out"=w479:errorcluster)  [unwired: 9 in]
          }
          frame "Documentation..." {
            n197 = call-poly <vilib>:"Open URL in Default Browser.vi"("error in (no error)"=w482, "URL"="https://astemes.github.io/astemes-lunit/") -> ("error out"=w483:errorcluster)  [unwired: 4 in, 1 out]
          }
          frame "Report issue..." {
            n198 = call-poly <vilib>:"Open URL in Default Browser.vi"("error in (no error)"=w486, "URL"="https://github.com/astemes/astemes-lunit/issues") -> ("error out"=w487:errorcluster)  [unwired: 4 in, 1 out]
          }
          frame "Post an Idea..." {
            n199 = call-poly <vilib>:"Open URL in Default Browser.vi"("error in (no error)"=w490, "URL"="https://www.vipm.io/post/suggestion/?package_name=astemes_lib_lunit&return_url=/package/astemes_lib_lunit/") -> ("error out"=w491:errorcluster)  [unwired: 4 in, 1 out]
          }
          frame "About" {
            n200 = call "About Dialog.vi"() -> ()  [unwired: 12 in]
          }
          frame "Exit" {
            n201 = call-dynamic "Stop.vi"("error in (no error)"=w498, "Execution UI In"=w499) -> ("error out"=w497:errorcluster, "Execution UI Out"=w496:refnum<class "Execution UI.lvclass">)  [unwired: 8 in]
          }
        }
      }
      event User Event {
        n202 = event-data() -> ()  [unwired: 1 in, 4 out]
      }
      event Panel Close? {
        w507 = TRUE  # Discard?
        n203 = event-data() -> ()  [unwired: 1 in, 4 out]
        n204 = call-dynamic "Stop.vi"("error in (no error)"=w503, "Execution UI In"=w506) -> ("error out"=w504:errorcluster, "Execution UI Out"=w505:refnum<class "Execution UI.lvclass">)  [unwired: 8 in]
        n205 = event-data ("Event Filter Node")("Discard?"=w507) -> ()  [unwired: 1 in, 1 out]
      }
    }
  }
  n206 = Unregister For Events(event registration refnum=w10, error in=w7) -> (error out=w6:errorcluster)
  n207 = Merge Errors(w6, w8) -> (w5:errorcluster)
  n208 = call <vilib>:"Clear Errors.vi"("error in (no error)"=w5) -> ()  [unwired: 5 in, 2 out]
